vi "create group specification.vi"(8 "error in":errorcluster, 10 "group data dictionary in":refnum<class "data bus dictionary.lvclass">, 11 "main data dictionary in":refnum<class "data bus dictionary.lvclass">) -> (0 "error out":errorcluster, 1 "group specification":T1[](array[typedef]), 2 "group data dictionary out":refnum<class "data bus dictionary.lvclass">, 3 "main data dictionary out":refnum<class "data bus dictionary.lvclass">)   [LabVIEW 2013, in "data bus dictionary.lvclass"]
doc: "Uses two data dictionaries and a set of tag names and types to create a group specification. This group specification is a special case of the transfer specification, and can be used to move data from one table to another table. These tables must share the same tags."
uses:
  data bus dictionary.lvclass
  tag/Data Type.ctl
  tag/data bus tag description.lvclass
  table/group specification.ctl
  table/data bus values.lvlib
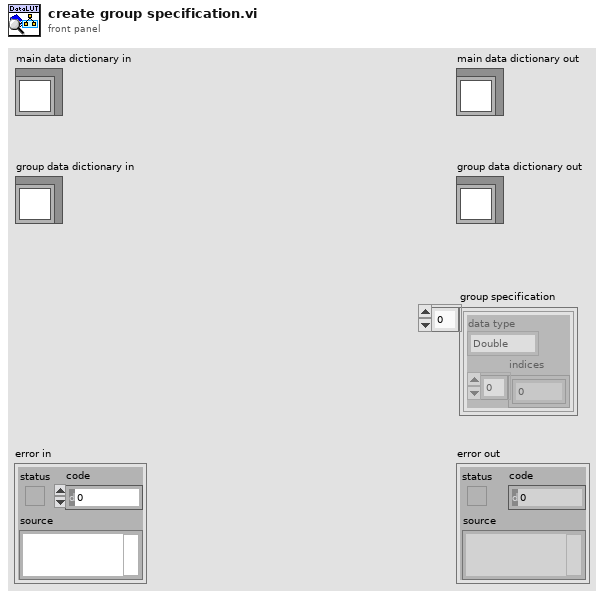
[diagram p1: front panel]
types:
  T1 = typedef "data bus values.lvlib/group specification.ctl" = cluster{"data type":T2, "indices":i32[]}
  T2 = typedef "data bus tag description.lvclass/Data Type.ctl" = enum16{"Double", "I64", "Boolean", "Array of Double", "Array of I64", "Variant"}
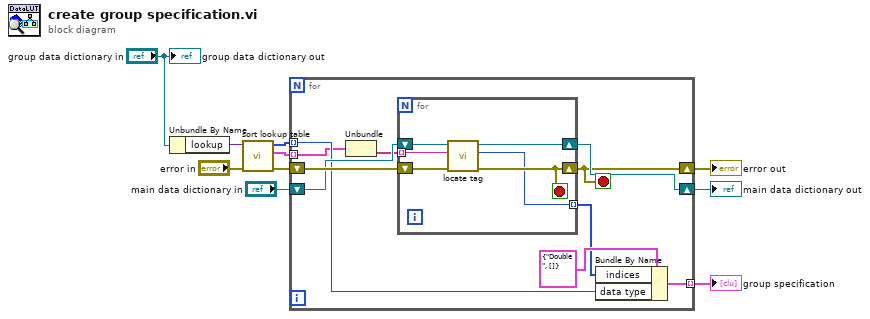
[diagram p0: block diagram]
diagram:
  n1 = Unbundle By Name("group data dictionary in") -> ("lookup"=w4:variant)
  n2 = call "sort lookup table.vi"("error in (no error)"="error in", "lookup"=w4) -> ("error out"=w3:errorcluster, "tags by type"=w1:cluster{"indices":i32[], "names":string[]}[], "types"=w2:T2[])  [unwired: 7 in]
  n3 = for {
    shift-right: [w18] -> w9
    shift-left: "main data dictionary in" -> [w19]
    shift-right: [w16] -> w7
    shift-left: w3 -> [w20]
    tunnel: [w17] -> w6 mode=indexing
    tunnel: w2 -> [w15] mode=indexing
    tunnel: w1 -> [w14] mode=indexing
    stop <- w16 stop-if-true
    n4 = Unbundle(w14) -> ("names"=w13:string[])  [unwired: 1 out]
    n5 = for {
      shift-right: [w24] -> w18
      shift-left: w19 -> [w26]
      tunnel: w13 -> [w21] mode=indexing
      shift-right: [w23] -> w16
      shift-left: w20 -> [w25]
      tunnel: [w22] -> w11 mode=indexing
      stop <- w23 stop-if-true
      n6 = call "locate tag.vi"("error in"=w25, "name"=w21, "data dictionary in"=w26) -> ("error out"=w23:errorcluster, "index"=w22:i32, "data dictionary out"=w24:refnum<class "data bus dictionary.lvclass">)  [unwired: 5 in, 1 out]
    }
    n7 = Bundle By Name(cluster=T1 {"data type"=enum."Double", "indices"=[]} ("group specification"), "indices"=w11, "data type"=w15) -> (w17:T1)
  }
  "error out" <- w7
  "main data dictionary out" <- w9
  "group specification" <- w6
  "group data dictionary out" <- "group data dictionary in"
